vi "set.vi"(9 "values":string[](array[string])=["0", "hola", "3,25"], 10 "variables":string[](array[string])=["intin", "strinin", "time"], 11 "Experience ID":string="Test") -> (0 "error out":errorcluster={"status"=TRUE, "code"=1, "source"="Bad condversion\nWhile writing variable: intin\nOn expID:Test"})   [LabVIEW 2014]
panel:
  # "Set"
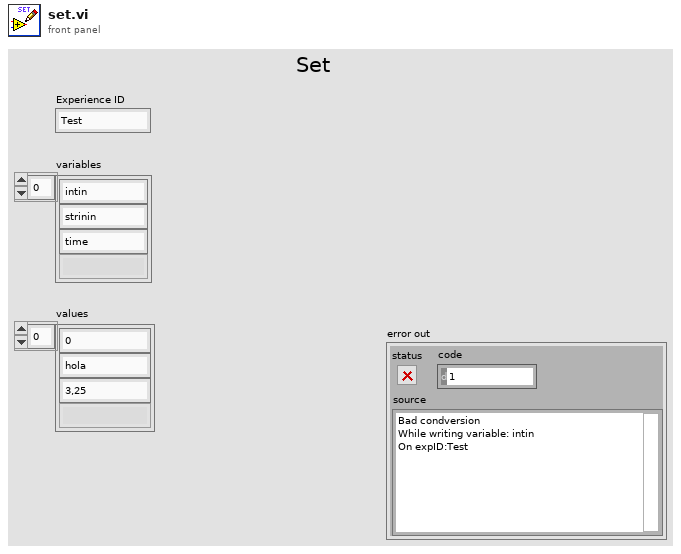
[diagram p1: front panel]
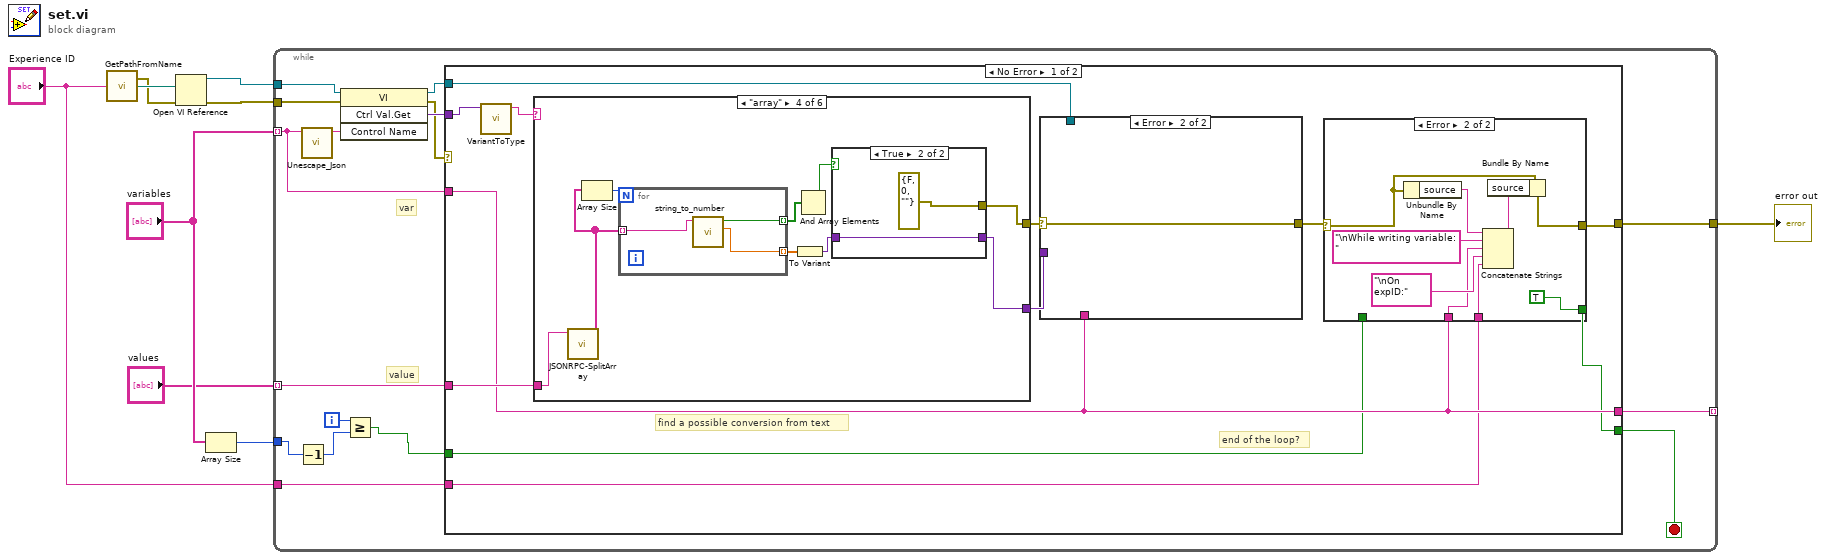
[diagram p0: block diagram]
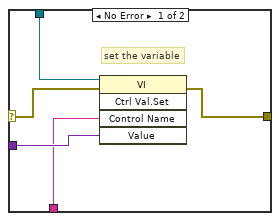
[diagram p3: hidden frame]
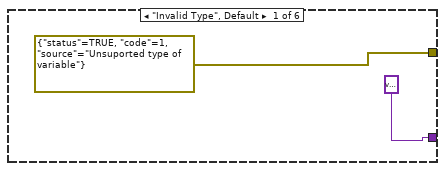
[diagram p4: hidden frame]
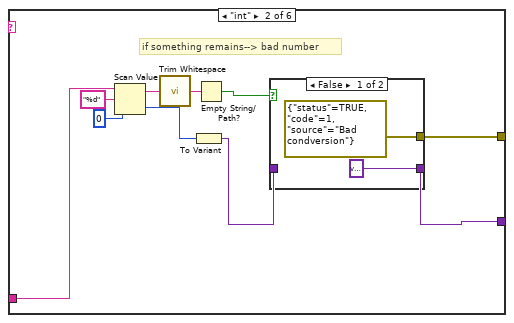
[diagram p5: hidden frame]
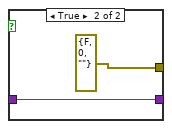
[diagram p6: hidden frame]
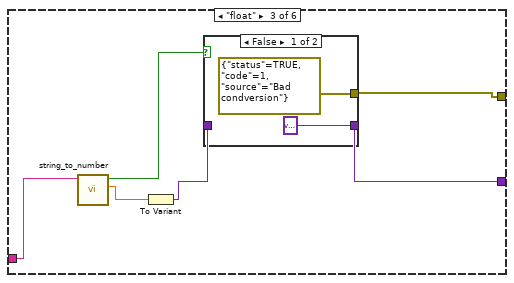
[diagram p7: hidden frame]
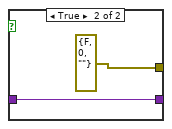
[diagram p8: hidden frame]
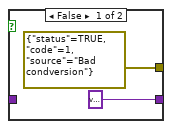
[diagram p9: hidden frame]
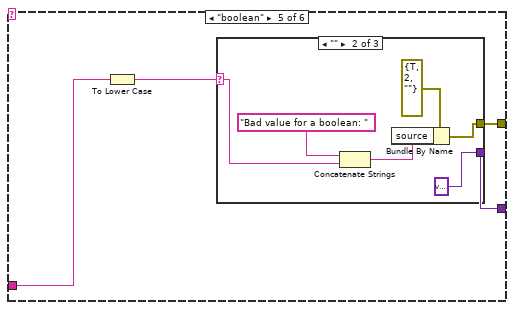
[diagram p10: hidden frame]
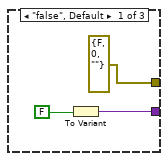
[diagram p11: hidden frame]
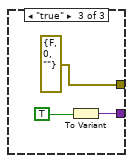
[diagram p12: hidden frame]
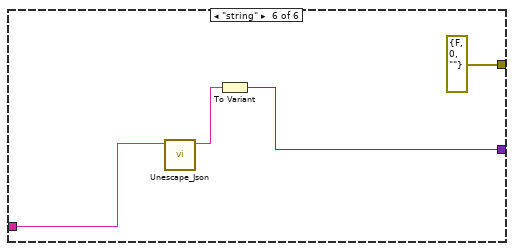
[diagram p13: hidden frame]
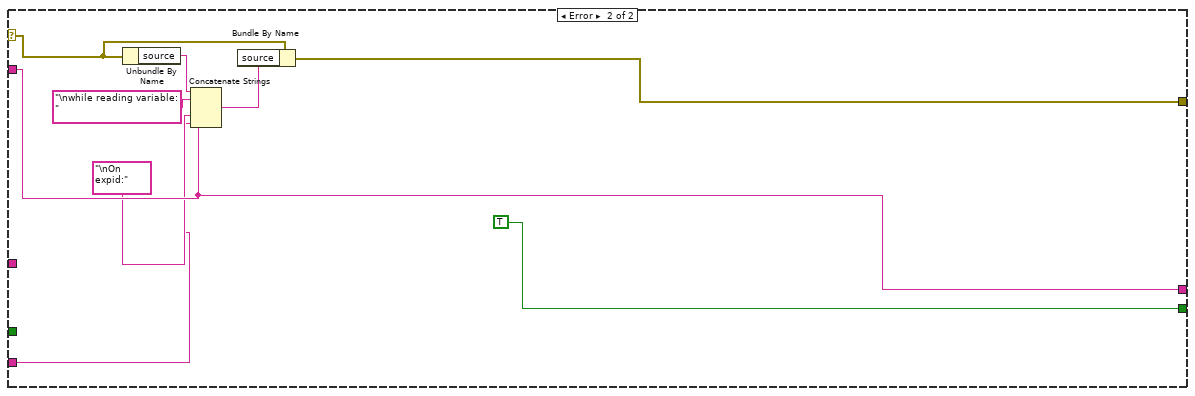
[diagram p14: hidden frame]
diagram:
  n1 = call "GetPathFromName.vi"("Experience ID"="Experience ID") -> ("Error out"=w8:errorcluster, "VI_Path"=w9:path)
  n2 = Open VI Reference(vi path=w9, error in (no error)=w8) -> (vi reference=w2:refnum<vi>, error out=w5:errorcluster)  [unwired: 1 in, 3 out]
  n3 = Array Size(array="variables") -> (size(s)=w6:i32)
  n4 = while {
    tunnel: "variables" -> [w10] mode=indexing
    tunnel: w2 -> [w25]
    tunnel: w6 -> [w17]
    tunnel: w5 -> [w24]
    tunnel: [w20] -> w1
    tunnel: [w19] -> _ mode=indexing
    tunnel: "Experience ID" -> [w18]
    tunnel: "values" -> [w13] mode=indexing
    i -> [w15]
    stop <- w21 stop-if-true
    # "value"
    # "var"
    n5 = Decrement(x=w17) -> (x-1=w14:i32)
    n6 = call "Unescape_Json.vi"("Json_String"=w10) -> ("String"=w11:string)  [unwired: 9 in]
    n7 = invoke class="VI" method="Ctrl Val.Get"(reference=w25, error in=w24, "Control Name"=w11) -> (reference out=w12:refnum<vi>, error out=w22:errorcluster, "Get Control Value Variant"=w23:variant)  [unwired: 1 in, 1 out]
    n8 = Greater Or Equal?(x=w15, y=w14) -> (x >= y?=w16:bool)
    n9 = case shown="No Error" w22 {
      selector: w22 -> [_ w124]
      tunnel: w23 -> [w27 _]
      tunnel: w16 -> [w28 _]
      tunnel: [w29 TRUE] -> w21
      tunnel: w10 -> [w33 w119]
      tunnel: [w30 w120] -> w20
      tunnel: [w33 w119] -> w19
      tunnel: w18 -> [w32 w117]
      tunnel: w13 -> [w36 _]
      tunnel: w12 -> [w34 _]
      frame No Error {
        # "end of the loop?"
        # "find a possible conversion from text"
        n10 = call "VariantToType.vi"("Variant"=w27) -> ("type Name"=w26:string)  [unwired: 10 in]
        n11 = case shown="\"array\"" w26 {
          tunnel: [errorcluster {"status"=TRUE, "code"=1, "source"="Unsuported type of variable"} ("error out") w59 w75 w82 w99 errorcluster {"status"=FALSE, "code"=0, "source"=""} ("error IO")] -> w37
          tunnel: w36 -> [_ w66 w76 w88 w97 w113]
          tunnel: [variant ("Variant") w61 w74 w81 w100 w116] -> w35
          frame "Invalid Type", Default {
          }
          frame "int" {
            # "if something remains--> bad number"
            n12 = Scan Value(string=w66, format string="%d", default (0 dbl)=0) -> (output string=w57:string, value=w63:i32)
            n13 = call <vilib>:"Trim Whitespace.vi"("string"=w57) -> ("trimmed string"=w58:string)  [unwired: 1 in]
            n14 = To Variant(anything=w63) -> (Variant=w60:variant)
            n15 = Empty String/Path?(string/path=w58) -> (empty?=w62:bool)
            n16 = case shown="False" w62 {
              tunnel: [variant w70] -> w61
              tunnel: w60 -> [_ w70]
              tunnel: [errorcluster {"status"=TRUE, "code"=1, "source"="Bad condversion"} ("error IO") errorcluster {"status"=FALSE, "code"=0, "source"=""} ("error IO")] -> w59
              frame False {
              }
              frame True {
              }
            }
          }
          frame "float" {
            n17 = call "string_to_number.vi"("String"=w76) -> ("default (0 dbl)"=w71:dbl, "conversionOK"=w73:bool)  [unwired: 9 in]
            n18 = To Variant(anything=w71) -> (Variant=w72:variant)
            n19 = case shown="False" w73 {
              tunnel: [variant w80] -> w74
              tunnel: w72 -> [_ w80]
              tunnel: [errorcluster {"status"=TRUE, "code"=1, "source"="Bad condversion"} ("error IO") errorcluster {"status"=FALSE, "code"=0, "source"=""} ("error IO")] -> w75
              frame False {
              }
              frame True {
              }
            }
          }
          frame "array" {
            n20 = call "JSONRPC-SplitArray.vi"("input string"=w88) -> ("array"=w86:string[])  [unwired: 10 in]
            n21 = Array Size(array=w86) -> (size(s)=w87:i32)
            n22 = for {
              N: w87 -> [_]
              tunnel: w86 -> [w92] mode=indexing
              tunnel: [w91] -> w84 mode=indexing
              tunnel: [w90] -> w85 mode=indexing
              n23 = call "string_to_number.vi"("String"=w92) -> ("default (0 dbl)"=w90:dbl, "conversionOK"=w91:bool)  [unwired: 9 in]
            }
            n24 = To Variant(anything=w85) -> (Variant=w89:variant)
            n25 = And Array Elements(Boolean array=w84) -> (logical AND=w83:bool)
            n26 = case shown="True" w83 {
              tunnel: [variant w96] -> w81
              tunnel: w89 -> [_ w96]
              tunnel: [errorcluster {"status"=TRUE, "code"=1, "source"="Bad condversion"} ("error IO") errorcluster {"status"=FALSE, "code"=0, "source"=""} ("error IO")] -> w82
              frame False {
              }
              frame True {
              }
            }
          }
          frame "boolean" {
            n27 = To Lower Case(string=w97) -> (all lower case string=w98:string)
            n28 = case shown="\"\"" w98 {
              selector: w98 -> [_ w107 _]
              tunnel: [w102 variant ("Variant") w112] -> w100
              tunnel: [errorcluster {"status"=FALSE, "code"=0, "source"=""} ("error IO") w105 errorcluster {"status"=FALSE, "code"=0, "source"=""} ("error IO")] -> w99
              frame "false", Default {
                n29 = To Variant(anything=FALSE) -> (Variant=w102:variant)
              }
              frame "" {
                n30 = Concatenate Strings("Bad value for a boolean: " ("source"), w107) -> (w109:string)
                n31 = Bundle By Name(cluster=errorcluster {"status"=TRUE, "code"=2, "source"=""} ("error IO"), "source"=w109) -> (w105:errorcluster)
              }
              frame "true" {
                n32 = To Variant(anything=TRUE) -> (Variant=w112:variant)
              }
            }
          }
          frame "string" {
            n33 = call "Unescape_Json.vi"("Json_String"=w113) -> ("String"=w114:string)  [unwired: 9 in]
            n34 = To Variant(anything=w114) -> (Variant=w116:variant)
          }
        }
        n35 = case shown="Error" w37 {
          selector: w37 -> [w52 w54]
          tunnel: [w51 w54] -> w31
          tunnel: w33 -> [w49 _]
          tunnel: w35 -> [w50 _]
          tunnel: w34 -> [w53 _]
          frame No Error {
            # "set the variable"
            n36 = invoke class="VI" method="Ctrl Val.Set"(reference=w53, error in=w52, "Control Name"=w49, "Value"=w50) -> (error out=w51:errorcluster)  [unwired: 1 in, 4 out]
          }
          frame Error {
          }
        }
        n37 = case shown="Error" w31 {
          selector: w31 -> [w39 w46]
          tunnel: [w39 w47] -> w30
          tunnel: [w38 TRUE] -> w29
          tunnel: w33 -> [_ w41]
          tunnel: w32 -> [_ w40]
          tunnel: w28 -> [w38 _]
          frame No Error {
            # "ok"
          }
          frame Error {
            n38 = Unbundle By Name(w46) -> ("source"=w45:string)
            n39 = Concatenate Strings(w45, "\nWhile writing variable: " ("string"), w41, "\nOn expID:" ("string"), w40) -> (w43:string)
            n40 = Bundle By Name(cluster=w46, "source"=w43) -> (w47:errorcluster)
          }
        }
      }
      frame Error {
        n41 = Unbundle By Name(w124) -> ("source"=w123:string)
        n42 = Concatenate Strings(w123, "\nwhile reading variable: " ("string"), w119, "\nOn expid:", w117) -> (w121:string)
        n43 = Bundle By Name(cluster=w124, "source"=w121) -> (w120:errorcluster)
      }
    }
  }
  "error out" <- w1
